vi "freqout --section -- format.vi"(4 "time (min)":dbl=nan, 5 "Magn Field (T)":dbl, 6 "delta freq":dbl, 7 "freqout action":enum16{"header", "one line", "one"}(ring)=enum."one line", 8 "segments string":string="Segments:{}", 9 "timestamp":timestamp, 10 "temperature":dbl, 11 "lorentzian":T1={"A (VHz)"=-1.0311345636926572, "ω (Hz)"=-1.0311345636926572, "Γ (Hz)"=-1.0311345636926572, "φ (rad)"=-1.0311345636926572, "Q"=-1.0311345636926572, "Norm  Ampl"=-1.0311345636926572, "z∞ (V)"=-1.0311345636926572+0.0i, "4corners"={"z (-pi/2)"=-1.0311345636926572+0.5736824521422934i, "z(inf)"=-0.5200164984937075+1.0975277942502903i, "z (pi/2)"=-1.0311345636926572+0.5736824521422934i, "z center"=-0.5136528600391839+0.580046090596817i, "z(0)"=-0.5200164984937075+1.0975277942502903i, "radius"=-1.0311345636926572}} {"z∞ (V)" format="%#_4p"; "Q" format="%#_4p"; "φ (rad)" format="%#_3p"; "Γ (Hz)" format="%#_5p"; "ω (Hz)" format="%#_9p"; "A (VHz)" format="%#_3p"}) -> (0 "output string":string)   [LabVIEW 2021]
uses:
  lorentzian.ctl
  circle corners.ctl
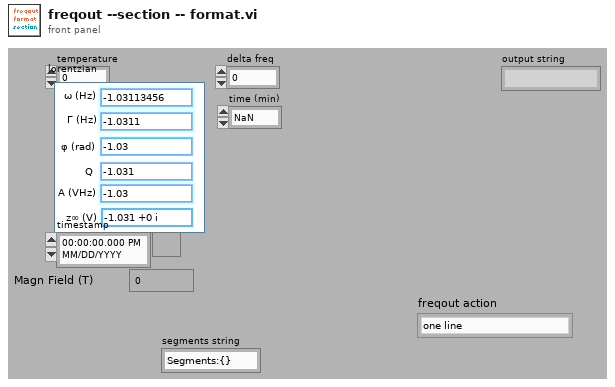
[diagram p1: front panel]
types:
  T1 = typedef "lorentzian.ctl" = cluster{"A (VHz)":dbl, "ω (Hz)":dbl, "Γ (Hz)":dbl, "φ (rad)":dbl, "Q":dbl, "Norm  Ampl":dbl, "z∞ (V)":cdb, "4corners":T2}
  T2 = typedef "circle corners.ctl" = cluster{"z (-pi/2)":cdb, "z(inf)":cdb, "z (pi/2)":cdb, "z center":cdb, "z(0)":cdb, "radius":dbl}
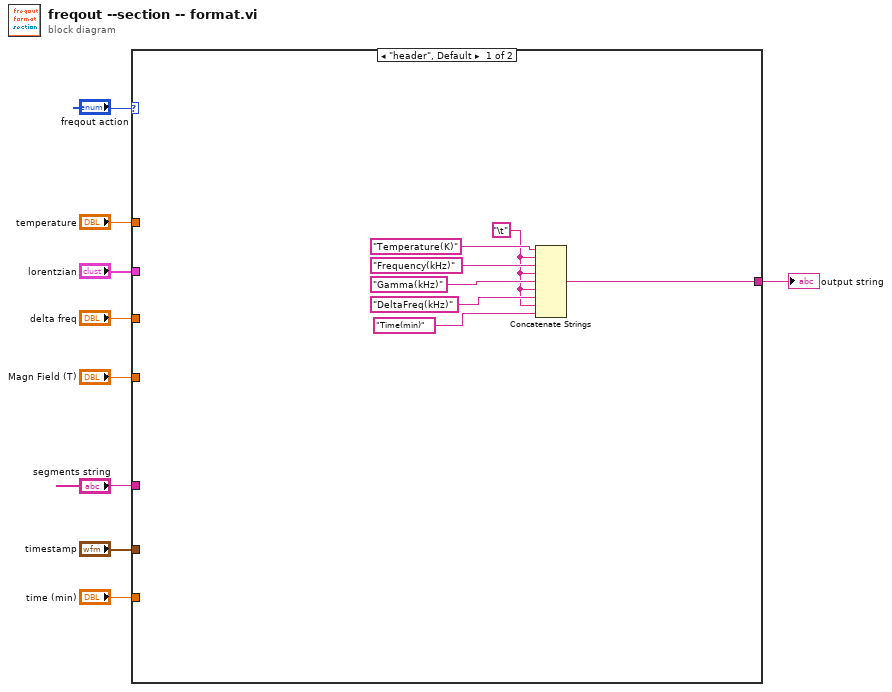
[diagram p0: block diagram]
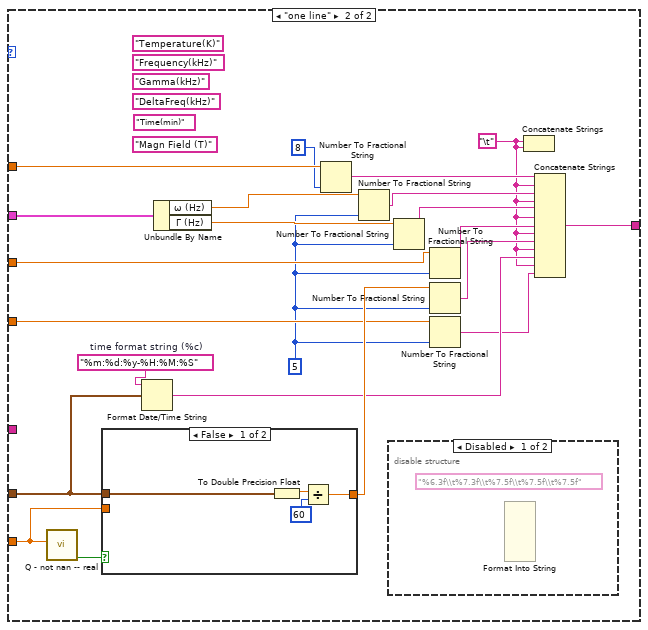
[diagram p2: hidden frame]
diagram:
  n1 = case shown="\"header\", Default" "freqout action" {
    tunnel: [w10 w29] -> w4
    tunnel: "segments string" -> [_ _]
    tunnel: "temperature" -> [_ w38]
    tunnel: "lorentzian" -> [_ w37]
    tunnel: "timestamp" -> [_ w23]
    tunnel: "delta freq" -> [_ w26]
    tunnel: "time (min)" -> [_ w24]
    tunnel: "Magn Field (T)" -> [_ w18]
    frame "header", Default {
      w12 = "\t"
      n2 = Concatenate Strings("Temperature(K)", w12, "Frequency(kHz)", w12, "Gamma(kHz)", w12, "DeltaFreq(kHz)", w12, "Time(min)") -> (w10:string)
    }
    frame "one line" {
      (unwired) "Magn Field (T)"
      w22 = "%m:%d:%y-%H:%M:%S"  # time format string (%c)
      (unwired) "Time(min)"
      (unwired) "DeltaFreq(kHz)"
      (unwired) "Gamma(kHz)"
      (unwired) "Frequency(kHz)"
      (unwired) "Temperature(K)"
      w20 = "\t"
      w17 = i16 5 ("precision (6)")
      n3 = call "Q - not nan -- real.vi"("Numeric"=w24) -> ("Boolean"=w25:bool)  [unwired: 9 in, 1 out]
      n4 = case shown="False" w25 {
        tunnel: w23 -> [w40 _]
        tunnel: [w39 w43] -> w28
        tunnel: w24 -> [_ w43]
        frame False {
          n5 = To Double Precision Float(number=w40) -> (double precision float=w42:dbl)
          n6 = Divide(x=w42, y=60) -> (x/y=w39:dbl)
        }
        frame True {
        }
      }
      n7 = Format Date/Time String(time format string (%c)=w22, seconds (now)=w23) -> (date/time string=w21:string)  [unwired: 1 in]
      n8 = Unbundle By Name(w37) -> ("ω (Hz)"=w35:dbl, "Γ (Hz)"=w33:dbl)
      n9 = Number To Fractional String(number=w38, precision (6)=i16 8) -> (F-format string=w36:string)  [unwired: 2 in]
      n10 = Number To Fractional String(number=w35, precision (6)=w17) -> (F-format string=w34:string)  [unwired: 2 in]
      n11 = disable-structure shown="Disabled" {
        frame Disabled {
          (unwired) "%6.3f\\t%7.3f\\t%7.5f\\t%7.5f\\t%7.5f"
          n12 = Format Into String() -> ()  [unwired: 8 in, 2 out]
        }
        frame Enabled {
        }
      }
      n13 = Number To Fractional String(number=w33, precision (6)=w17) -> (F-format string=w31:string)  [unwired: 2 in]
      n14 = Number To Fractional String(number=w26, precision (6)=w17) -> (F-format string=w32:string)  [unwired: 2 in]
      n15 = Number To Fractional String(number=w28, precision (6)=w17) -> (F-format string=w27:string)  [unwired: 2 in]
      n16 = Number To Fractional String(number=w18, precision (6)=w17) -> (F-format string=w19:string)  [unwired: 2 in]
      n17 = Concatenate Strings(w20, w20) -> ()  [unwired: 1 out]
      n18 = Concatenate Strings(w36, w20, w34, w20, w31, w20, w32, w20, w27, w20, w21, w20, w19) -> (w29:string)
    }
  }
  "output string" <- w4
